vi "Global_STOP.vi"() -> ()   [LabVIEW 2016]
panel:
  in  "STOP":bool
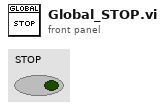
[diagram p1: front panel]
diagram:
